vi "PCAN.vi"() -> ()   [LabVIEW 2020]
uses:
  <userlib>/PCANBasic/ctl/TPCANStatus.ctl
  <userlib>/PCANBasic/ctl/TPCANMsgFD.ctl
  <userlib>/PCANBasic/PCANBasic.lvlib
panel:
  in  "停止 2":bool
  in  "停止":bool
  in  "继电器控制":T1
  out "TCANStatus":T2 items=["PCAN_ERROR_OK"=0, "PCAN_ERROR_XMTFULL"=1, "PCAN_ERROR_OVERRUN"=2, "PCAN_ERROR_BUSLIGHT"=4, "PCAN_ERROR_BUSHEAVY"=8, "PCAN_ERROR_BUSPASSIVE"=262144, "PCAN_ERROR_BUSOFF"=16, "PCAN_ERROR_QRCVEMPTY"=32, "PCAN_ERROR_QOVERRUN"=64, "PCAN_ERROR_QXMTFULL"=128, "PCAN_ERROR_REGTEST"=256, "PCAN_ERROR_NODRIVER"=512, "PCAN_ERROR_HWINUSE"=1024, "PCAN_ERROR_NETINUSE"=2048, "PCAN_ERROR_ILLHW"=5120, "PCAN_ERROR_ILLNET"=6144, "PCAN_ERROR_ILLCLIENT"=7168, "PCAN_ERROR_RESOURCE"=8192, "PCAN_ERROR_ILLPARAMTYPE"=16384, "PCAN_ERROR_ILLPARAMVAL"=32768, "PCAN_ERROR_UNKNOWN"=65536, "PCAN_ERROR_ILLDATA"=131072, "PCAN_ERROR_CAUTION"=33554432, "PCAN_ERROR_INITIALIZE"=67108864, "PCAN_ERROR_ILLOPERATION"=134217728]
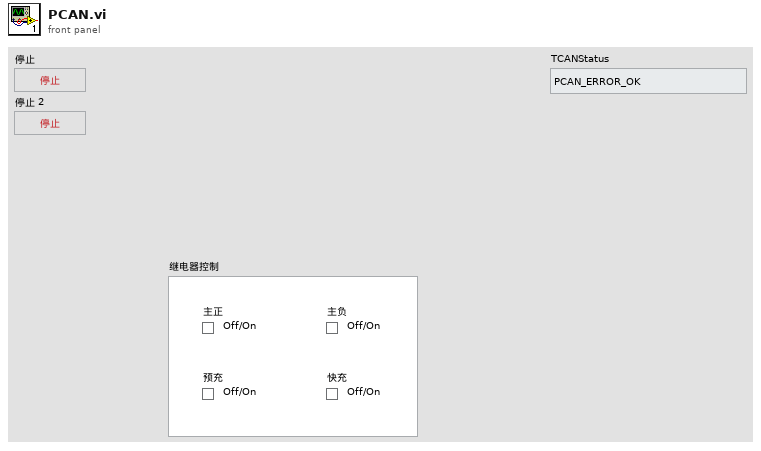
[diagram p1: front panel]
types:
  T1 = typedef "继电器控制.ctl" = cluster{"主正":bool, "主负":bool, "快充":bool, "预充":bool}
  T2 = typedef "PCANBasic.lvlib/TPCANStatus.ctl" = u32
  T3 = typedef "PCANBasic.lvlib/TPCANMsgFD.ctl" = cluster{"ID":u32, "MSGTYPE":u8, "DLC":u8, "DATA":cluster{"[0]":u8, "[1]":u8, "[2]":u8, "[3]":u8, "[4]":u8, "[5]":u8, "[6]":u8, "[7]":u8, "[8]":u8, "[9]":u8, "[10]":u8, "[11]":u8, "[12]":u8, "[13]":u8, "[14]":u8, "[15]":u8, "[16]":u8, "[17]":u8, "[18]":u8, "[19]":u8, "[20]":u8, "[21]":u8, "[22]":u8, "[23]":u8, "[24]":u8, "[25]":u8, "[26]":u8, "[27]":u8, "[28]":u8, "[29]":u8, "[30]":u8, "[31]":u8, "[32]":u8, "[33]":u8, "[34]":u8, "[35]":u8, "[36]":u8, "[37]":u8, "[38]":u8, "[39]":u8, "[40]":u8, "[41]":u8, "[42]":u8, "[43]":u8, "[44]":u8, "[45]":u8, "[46]":u8, "[47]":u8, "[48]":u8, "[49]":u8, "[50]":u8, "[51]":u8, "[52]":u8, "[53]":u8, "[54]":u8, "[55]":u8, "[56]":u8, "[57]":u8, "[58]":u8, "[59]":u8, "[60]":u8, "[61]":u8, "[62]":u8, "[63]":u8}}
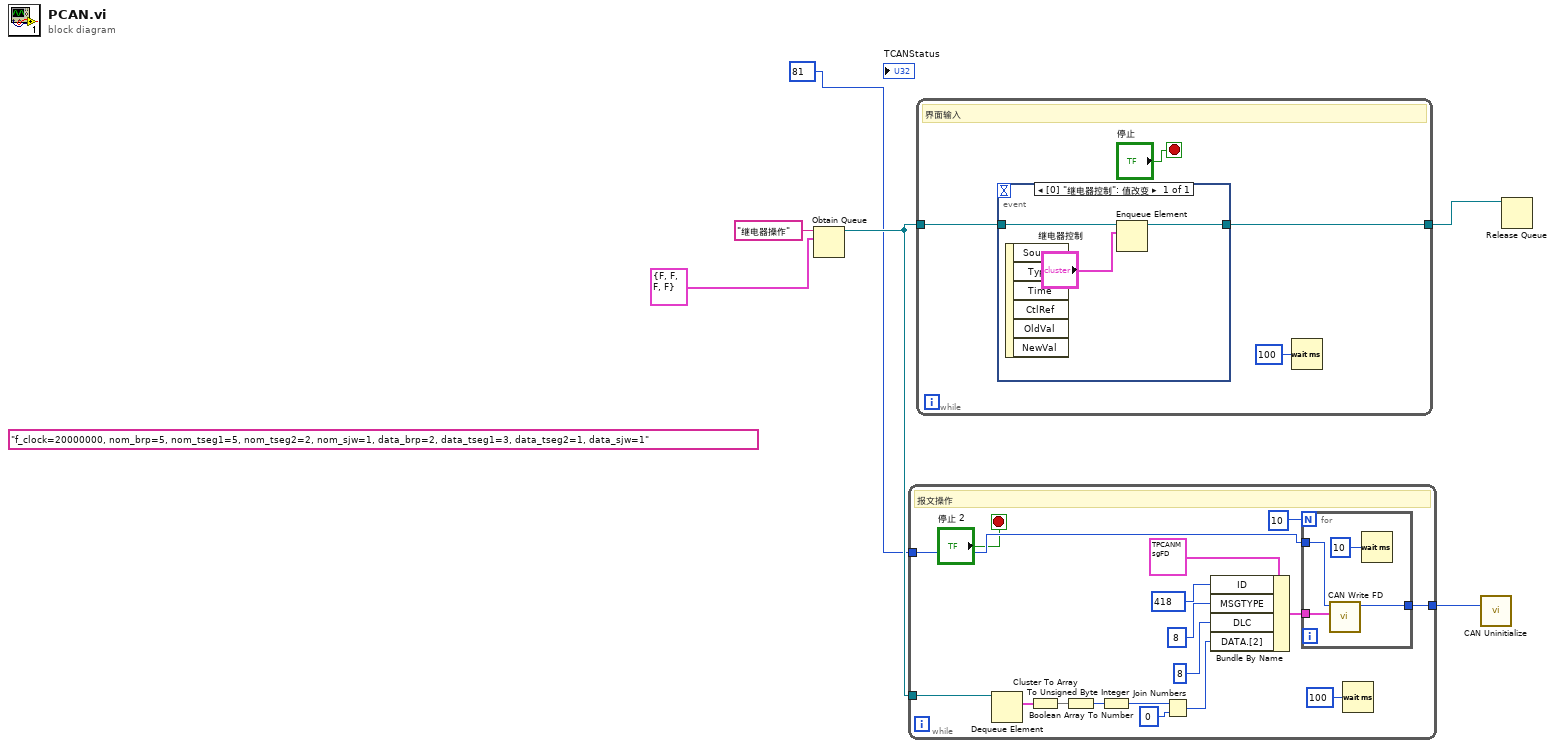
[diagram p0: block diagram]
diagram:
  (unwired) "f_clock=20000000, nom_brp=5, nom_tseg1=5, nom_tseg2=2, nom_sjw=1, data_brp=2, data_tseg1=3, data_tseg2=1, data_sjw=1" ("BitrateFD")
  n1 = Obtain Queue(name (unnamed)="继电器操作" ("名称（未命名）"), element data type=T1 {"主正"=FALSE, "主负"=FALSE, "快充"=FALSE, "预充"=FALSE} ("继电器控制")) -> (queue out=w3:refnum<queue>)  [unwired: 3 in, 2 out]
  n2 = while {
    tunnel: u16 81 ("Channel") -> [w12]
    tunnel: [w10] -> w5
    tunnel: w3 -> [w9]
    stop <- "停止 2" stop-if-true
    # "报文操作"
    n3 = Dequeue Element(queue=w9) -> (element=w23:T1)  [unwired: 2 in, 3 out]
    n4 = Cluster To Array(cluster=w23) -> (array=w22:bool[])
    n5 = Boolean Array To Number(Boolean array=w22) -> (number=w20:u32)
    n6 = To Unsigned Byte Integer(number=w20) -> (unsigned 8bit integer=w15:u8)
    n7 = Join Numbers(hi=w15, lo=u8 0) -> ((hi.lo)=w14:u16)
    n8 = Bundle By Name(cluster=T3 {"ID"=0, "MSGTYPE"=0, "DLC"=0, "DATA"={"[0]"=0, "[1]"=0, "[2]"=0, "[3]"=0, "[4]"=0, "[5]"=0, "[6]"=0, "[7]"=0, "[8]"=0, "[9]"=0, "[10]"=0, "[11]"=0, "[12]"=0, "[13]"=0, "[14]"=0, "[15]"=0, "[16]"=0, "[17]"=0, "[18]"=0, "[19]"=0, "[20]"=0, "[21]"=0, "[22]"=0, "[23]"=0, "[24]"=0, "[25]"=0, "[26]"=0, "[27]"=0, "[28]"=0, "[29]"=0, "[30]"=0, "[31]"=0, "[32]"=0, "[33]"=0, "[34]"=0, "[35]"=0, "[36]"=0, "[37]"=0, "[38]"=0, "[39]"=0, "[40]"=0, "[41]"=0, "[42]"=0, "[43]"=0, "[44]"=0, "[45]"=0, "[46]"=0, "[47]"=0, "[48]"=0, "[49]"=0, "[50]"=0, "[51]"=0, "[52]"=0, "[53]"=0, "[54]"=0, "[55]"=0, "[56]"=0, "[57]"=0, "[58]"=0, "[59]"=0, "[60]"=0, "[61]"=0, "[62]"=0, "[63]"=0}} ("MessageBuffer"), "ID"=u32 418, "MSGTYPE"=u8 8, "DLC"=u8 8, "DATA.[2]"=w14) -> (w13:T3)
    n9 = for {
      N: 10 -> [_]
      tunnel: w13 -> [w27]
      tunnel: w12 -> [w26]
      tunnel: [w24] -> w10
      n10 = call <userlib>:"CAN Write FD.vi"("MessageBuffer in"=w27, "Channel"=w26) -> ("TCANStatus"=w24:T2)  [unwired: 6 in, 3 out]
      n11 = Wait (ms)(milliseconds to wait=u32 10 ("等待时间（毫秒）")) -> ()  [unwired: 1 out]
    }
    n12 = Wait (ms)(milliseconds to wait=u32 100 ("等待时间（毫秒）")) -> ()  [unwired: 1 out]
  }
  n13 = while {
    tunnel: w3 -> [w31]
    tunnel: [w29] -> w2
    stop <- "停止" stop-if-true
    # "界面输入"
    n14 = event shown="[0] \"继电器控制\": 值改变" {
      selector: _ -> [_]
      dyn-events: _ -> [_]
      timeout: _ -> [_]
      tunnel: w31 -> [w34]
      tunnel: [w33] -> w29
      event Value Change {
        n15 = event-data() -> ()  [unwired: 1 in, 6 out]
        n16 = Enqueue Element(queue=w34, element="继电器控制") -> (queue out=w33:refnum<queue>)  [unwired: 2 in, 2 out]
      }
    }
    n17 = Wait (ms)(milliseconds to wait=u32 100 ("等待时间（毫秒）")) -> ()  [unwired: 1 out]
  }
  n18 = call <userlib>:"CAN Uninitialize.vi"("Channel"=w5) -> ()  [unwired: 10 in, 1 out]
  n19 = Release Queue(queue=w2) -> ()  [unwired: 2 in, 3 out]
